vi "Xsens FP1632 (SubVI).vi"(11 "6 Byte Hex String":string) -> (3 "DBL":dbl)   [LabVIEW 2019]
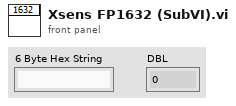
[diagram p1: front panel]
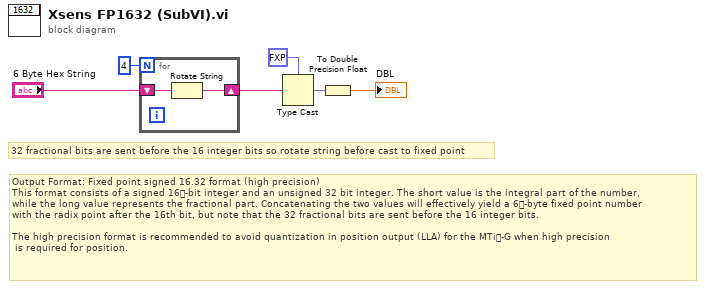
[diagram p0: block diagram]
diagram:
  # "32 fractional bits are sent before the 16 integer bits so rotate string before cast to fixed point"
  # "Output Format: Fixed point signed 16.32 format (high precision)\nThis format consists of a signed 16-bit integer and an unsigned 32 bit integer. The short value is the integral part of the number, \nwhile the long value represents the fractional part. Concatenating the two values will effectively yield a 6-byte fixed point number \nwith the radix point after the 16th bit, but note that the 32 fractional bits are sent before the 16 integer bits.\n\nThe high precision format is recommended to avoid quantization in position output (LLA) for the MTi-G when high precision\n is required for position."
  n1 = for {
    N: 4 -> [_]
    shift-right: [w7] -> w5
    shift-left: "6 Byte Hex String" -> [w8]
    n2 = Rotate String(1:w8) -> (0:w7:string)
  }
  n3 = Type Cast(type=fxp<+/-,48,16> 0.0 ("fixed-point"), x=w5) -> (*(type *) &x=w3:fxp<+/-,48,16>)
  n4 = To Double Precision Float(number=w3) -> (double precision float=→"DBL":dbl)
